vi "PicoScope6000SetDataBufferBulk.vi"(5 "enabled array":i16[](array[numeric]), 7 "Buffer and Transfer Settings":T3 {"Down-Sample Mode" items=["None", "Aggregate", "Decimate", "Average"]; "Down Sample Ratio" step=1; "Samples" format="%_6p"}, 8 "error in (no error)":errorcluster, 9 "Device Info":T1, 10 "Data Pointers In":T2, 11 "handle in":i16) -> (0 "error out":errorcluster, 3 "handle out":i16)   [LabVIEW 2009]
doc: "Calls SetDataBuffers, and assigns Pico buffers"
uses:
  ps6000.dll
  shared/PicoBuffers.ctl
  shared/Buffer and Transfer Settings.ctl
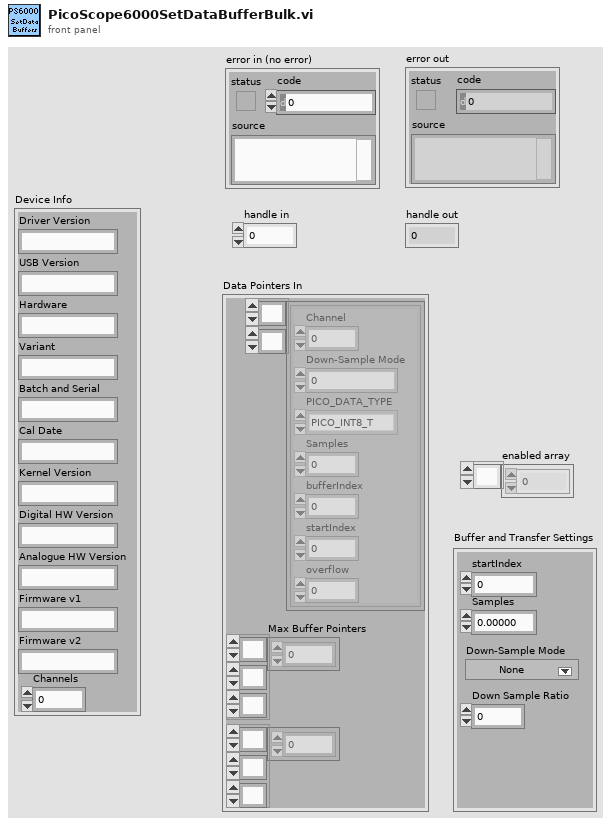
[diagram p1: front panel]
types:
  T1 = cluster{"Driver Version":string, "USB Version":string, "Hardware":string, "Variant":string, "Batch and Serial":string, "Cal Date":string, "Kernel Version":string, "Digital HW Version":string, "Analogue HW Version":string, "Firmware v1":string, "Firmware v2":string, "Channels":i16}
  T2 = typedef "PicoBuffers.ctl" = cluster{"Max Buffer Pointers":u64[][][], "Min Buffer Pointers":u64[][][], "StreamingDataInfo":cluster{"Channel":u32, "Down-Sample Mode":u32, "PICO_DATA_TYPE":enum32{"PICO_INT8_T", "PICO_INT16_T", "PICO_INT32_T", "PICO_UINT32_T", "PICO_INT64_T", ""}, "Samples":i32, "bufferIndex":u64, "startIndex":i32, "overflow":i16}[][]}
  T3 = typedef "Buffer and Transfer Settings.ctl" = cluster{"startIndex":u64, "Samples":u64, "Down Sample Ratio":u64, "Down-Sample Mode":u32}
  T4 = cluster{"status":bool, "code":u32, "source":string}
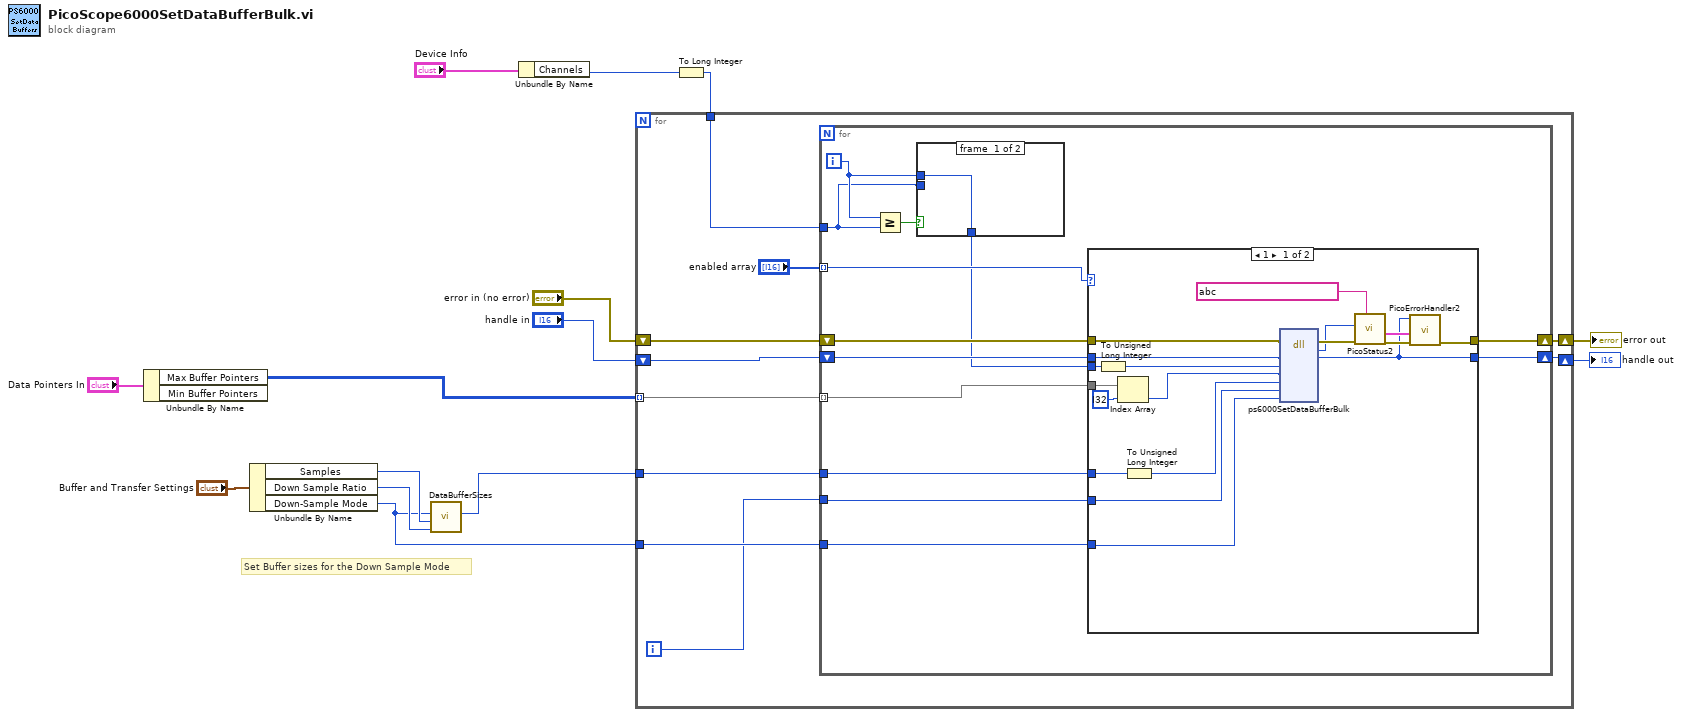
[diagram p0: block diagram]
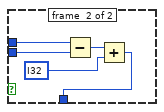
[diagram p2: hidden frame]
diagram:
  # "Set Buffer sizes for the Down Sample Mode"
  n1 = Unbundle By Name("Data Pointers In") -> ("Max Buffer Pointers"=w4:u64[][][])  [unwired: 1 out]
  n2 = Unbundle By Name("Buffer and Transfer Settings") -> ("Samples"=w6:u64, "Down Sample Ratio"=w7:u64, "Down-Sample Mode"=w5:u32)
  n3 = call "DataBufferSizes.vi"("Down Sample Ratio"=w7, "Number of Samples"=w6, "Down-Sample Mode"=w5) -> ("Max Buffer Size"=w8:i32)  [unwired: 7 in, 1 out]
  n4 = Unbundle By Name("Device Info") -> ("Channels"=w2:i16)
  n5 = To Long Integer(number=w2) -> (32bit integer=w3:i32)
  n6 = for {
    tunnel: w8 -> [w20]
    tunnel: w5 -> [w19]
    tunnel: w4 -> [w18] mode=indexing
    shift-right: [w24] -> w13
    shift-left: "error in (no error)" -> [w22]
    shift-right: [w23] -> w12
    shift-left: "handle in" -> [w21]
    tunnel: w3 -> [w15]
    i -> [w16]
    n7 = for {
      tunnel: w19 -> [w37]
      tunnel: w20 -> [w34]
      tunnel: "enabled array" -> [w27] mode=indexing
      tunnel: w18 -> [w33] mode=indexing
      shift-right: [w32] -> w24
      shift-left: w22 -> [w36]
      shift-right: [w31] -> w23
      shift-left: w21 -> [w35]
      tunnel: w16 -> [w25]
      tunnel: w15 -> [w28]
      i -> [w29]
      n8 = Greater Or Equal?(x=w29, y=w28) -> (x >= y?=w30:bool)
      n9 = case shown="True" w30 {
        tunnel: [w38 w42] -> w26
        tunnel: w28 -> [_ w41]
        tunnel: w29 -> [w38 w40]
        frame #0 {
        }
        frame #1 {
          n10 = Subtract(x=w40, y=w41) -> (x-y=w39:i32)
          n11 = Add(x=w39, y=i32 ?) -> (x+y=w42:i32)
        }
      }
      n12 = case shown="1" w27 {
        tunnel: w26 -> [w60 _]
        tunnel: w36 -> [w57 w63]
        tunnel: w35 -> [w56 w62]
        tunnel: w37 -> [w53 _]
        tunnel: [w47 w63] -> w32
        tunnel: [w46 w62] -> w31
        tunnel: w34 -> [w61 _]
        tunnel: w33 -> [w58 _]
        tunnel: w25 -> [w44 _]
        frame #0 {
          n13 = To Unsigned Long Integer(number=w60) -> (unsigned 32bit integer=w55:u32)
          n14 = Index Array(array=w58, index=i32 ?) -> (element=w54:u64)
          n15 = To Unsigned Long Integer(number=w61) -> (unsigned 32bit integer=w52:u32)
          n16 = dll-call lib="PS6000.dll" fn="ps6000SetDataBufferBulk" ("ps3000.dll:_ps3000_open_unit@0")(error in=w57, "handle"=w56, "channel"=w55, "bufferMax"=w54, "bufferLth"=w52, "waveform"=w44, "downSampleRatioMode"=w53) -> (error out=w49:errorcluster, "PICO_STATUS"=w48:u32, "handle"=w46:i16)  [unwired: 7 in, 1 out]
          n17 = call "PicoStatus2.vi"("PICO source"=string ? ("source"), "Error in"=w49, "PICO STATUS"=w48) -> ("error out"=w51:errorcluster, "PICO_STATUS out"=w50:T4)  [unwired: 5 in]
          n18 = call "PicoErrorHandler2.vi"("error in (no error)"=w51, "PICO_STATUS in"=w50, "handle In"=w46) -> ("error out"=w47:errorcluster)  [unwired: 8 in]
        }
        frame #1 {
        }
      }
    }
  }
  "error out" <- w13
  "handle out" <- w12
